vi "Read TOML File (LV).vi"(7 "Default Value":variant, 8 "error in (no error)":errorcluster, 9 "Error if missing element":bool caption="Error if missing element (F)", 11 "file path (use dialog)":path) -> (0 "error out":errorcluster, 2 "Missing elements":string[](array[string]), 3 "Value":variant)   [LabVIEW 2020, in "TOML.lvlib"]
doc: "This VI is kept to maintain compatibility with older versions but it's recommended to use the vim instead"
uses:
  TOML.lvlib
  22b0ca1a-c345-4be7-a7a8-e1286971195a.vi
  TOML to LabVIEW.vi
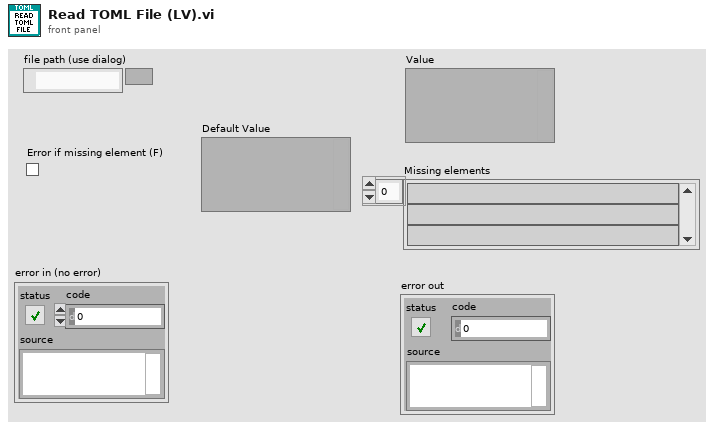
[diagram p1: front panel]
types:
  T1 = enum16{"open", "replace", "create", "open or create", "replace or create", "replace or create with confirmation"}
  T2 = typedef "TOML.lvlib/TOML Value.ctl" = cluster{"type":enum16{"Table", "Array", "String", "Integer", "Float", "Boolean", "Offset Date-Time", "Local Date-Time", "Local Date", "Local Time", "Path"}, "value":variant}
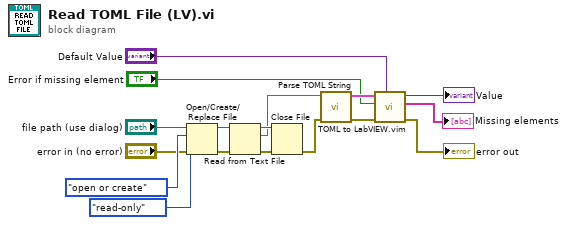
[diagram p0: block diagram]
diagram:
  n1 = Open/Create/Replace File(file path (use dialog)="file path (use dialog)", error in="error in (no error)", operation (0:open)=T1."open or create", access (0:read/write)=enum16{"read/write", "read-only", "write-only"}."read-only") -> (refnum out=w14:refnum<file>, error out=w15:errorcluster)  [unwired: 2 in, 1 out]
  n2 = Read from Text File(file (use dialog)=w14, error in=w15) -> (refnum out=w12:refnum<file>, text=w10:string, error out=w13:errorcluster)  [unwired: 2 in, 1 out]
  n3 = Close File(refnum=w12, error in=w13) -> (error out=w9:errorcluster)  [unwired: 1 out]
  n4 = call "Parse TOML String.vi"("error in (no error)"=w9, "String"=w10) -> ("error out"=w5:errorcluster, "Value"=w7:T2)  [unwired: 8 in]
  n5 = call "TOML to LabVIEW.vim"("datatype"="Default Value", "error in (no error)"=w5, "Error if missing element"="Error if missing element", "Value"=w7) -> ("error out"=→"error out":errorcluster, "Missing elements"=→"Missing elements":string[], "LV Data"=→"Value":variant)  [unwired: 5 in]
